vi "_Delete.vi"(8 "error in":errorcluster, 11 "Device In":i32) -> (0 "error out":errorcluster)   [LabVIEW 2013]
uses:
  phidget21.dll
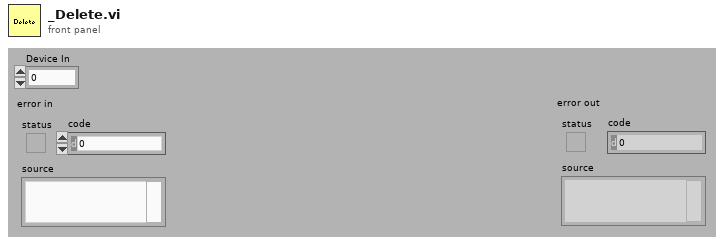
[diagram p1: front panel]
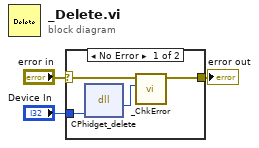
[diagram p0: block diagram]
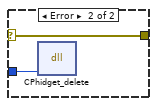
[diagram p2: hidden frame]
diagram:
  n1 = case shown="No Error" "error in" {
    selector: "error in" -> [w6 w9]
    tunnel: [w4 w9] -> w2
    tunnel: "Device In" -> [w7 w8]
    frame No Error {
      n2 = dll-call lib="phidget21.*" fn="CPhidget_delete"("phid"=w7) -> (w5:i32)  [unwired: 4 in, 2 out]
      n3 = call "_ChkError.vi"("Return Code"=w5, "error in (no error)"=w6) -> ("error out"=w4:errorcluster)  [unwired: 9 in]
    }
    frame Error {
      n4 = dll-call lib="phidget21.dll" fn="CPhidget_delete"("phid"=w8) -> ()  [unwired: 5 in, 2 out]
    }
  }
  "error out" <- w2
